vi "Offset XY Graph.vi"(8 "error in (no error)":errorcluster, 9 "y offset (0)":dbl, 10 "x offset (0)":dbl, 11 "graph_utilities in":refnum<class "graph_utilities.lvclass">) -> (0 "error out":errorcluster, 3 "graph_utilities out":refnum<class "graph_utilities.lvclass">)   [LabVIEW 2019, in "graph_utilities.lvclass"]
uses:
  graph_utilities.lvclass
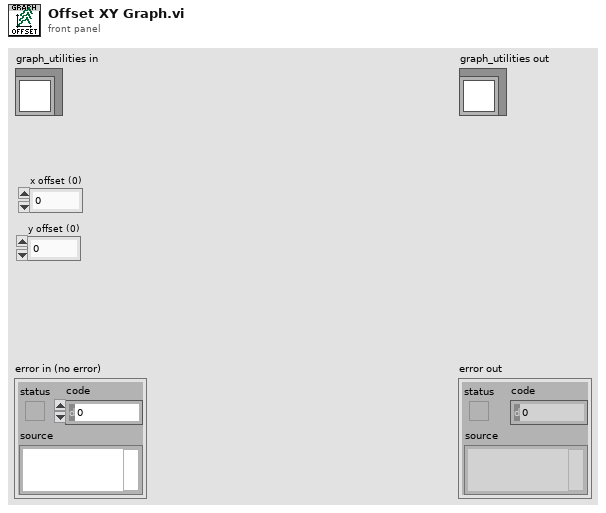
[diagram p1: front panel]
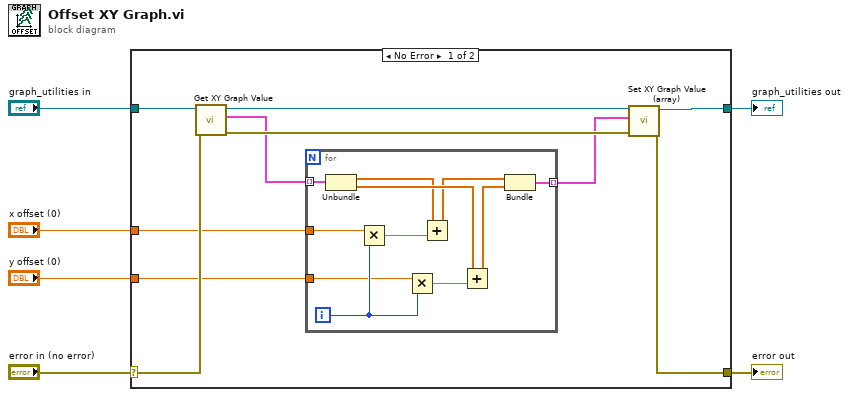
[diagram p0: block diagram]
diagram:
  n1 = case shown="No Error" "error in (no error)" {
    selector: "error in (no error)" -> [w13 w29]
    tunnel: [w12 w29] -> w5
    tunnel: [w14 w28] -> w3
    tunnel: "graph_utilities in" -> [w15 w28]
    tunnel: "y offset (0)" -> [w11 _]
    tunnel: "x offset (0)" -> [w10 _]
    frame No Error {
      n2 = call "Get XY Graph Value.vi"("error in (no error)"=w13, "graph_utilities in"=w15) -> ("error out"=w9:errorcluster, "Value"=w8:cluster{"X":dbl[], "Y":dbl[]}[], "graph_utilities out"=w16:refnum<class "graph_utilities.lvclass">)  [unwired: 7 in]
      n3 = for {
        tunnel: w11 -> [w19]
        tunnel: w10 -> [w25]
        tunnel: w8 -> [w24] mode=indexing
        tunnel: [w23] -> w7 mode=indexing
        i -> [w20]
        n4 = Unbundle(w24) -> ("X"=w18:dbl[], "Y"=w22:dbl[])
        n5 = Multiply(x=w25, y=w20) -> (x*y=w26:dbl)
        n6 = Multiply(x=w19, y=w20) -> (x*y=w27:dbl)
        n7 = Add(x=w18, y=w26) -> (x+y=w17:dbl[])
        n8 = Add(x=w22, y=w27) -> (x+y=w21:dbl[])
        n9 = Bundle(w17, w21) -> (w23:cluster{dbl[], dbl[]})  [unwired: 1 in]
      }
      n10 = call "Set XY Graph Value (array).vi"("error in (no error)"=w9, "Value"=w7, "graph_utilities in"=w16) -> ("error out"=w12:errorcluster, "graph_utilities out"=w14:refnum<class "graph_utilities.lvclass">)  [unwired: 7 in]
    }
    frame Error {
    }
  }
  "error out" <- w5
  "graph_utilities out" <- w3
